vi "Destroy.vi"(8 "error in":errorcluster, 11 "measurement service v1 in":refnum<class "Measurement Service V1.lvclass">) -> (0 "error out":errorcluster)   [LabVIEW 2020, in "Plug-In SDK Measurement.lvlib" / "Measurement Service V1.lvclass"]
uses:
  Measurement Service V1.lvclass
  Measurement Service V1.lvclass/Measurement Service V1.ctl
  gRPC/Generated APIs/ni/measurementlink/measurement/v1/RPC Service/MeasurementService/MeasurementServiceBaseV1.lvclass
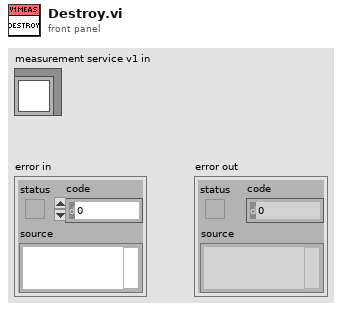
[diagram p1: front panel]
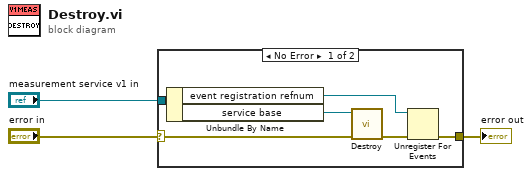
[diagram p0: block diagram]
diagram:
  n1 = case shown="No Error" "error in" {
    selector: "error in" -> [w8 w10]
    tunnel: [w6 w10] -> w2
    tunnel: "measurement service v1 in" -> [w9 _]
    frame No Error {
      n2 = Unbundle By Name(w9) -> ("event registration refnum"=w4:refnum<event-registration>, "service base"=w5:refnum<class "MeasurementServiceBaseV1.lvclass">)
      n3 = call-dynamic "Destroy.vi"("error in (no error)"=w8, "SignalGeneratorService in"=w5) -> ("error out"=w7:errorcluster)  [unwired: 8 in, 1 out]
      n4 = Unregister For Events(event registration refnum=w4, error in=w7) -> (error out=w6:errorcluster)
    }
    frame Error {
    }
  }
  "error out" <- w2
